vi "tsdiag_can_routine_control.vi"(6 "ATimeoutMS":i32, 8 "ARoutintID":u16, 9 "ARoutineControlType":u8, 10 "ADiagModuleIndex":i32, 11 "路径输入":path) -> (2 "返回类型":i32, 3 "路径输出":path)   [LabVIEW 2019]
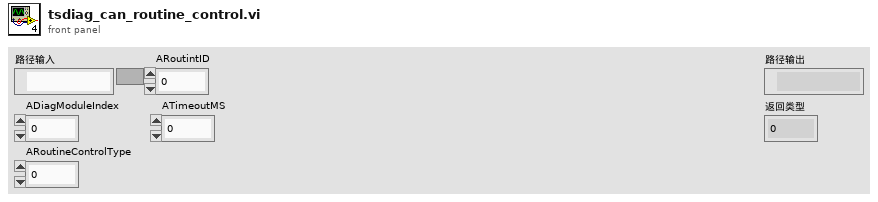
[diagram p1: front panel]
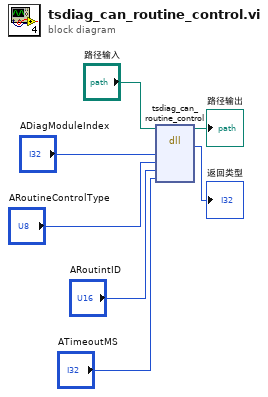
[diagram p0: block diagram]
diagram:
  n1 = dll-call lib="C:/Users/XYY/Desktop/LabView Demo/TSCAN_LB2018_V1.4_20220309/Config/TSMaster.dll" fn="tsdiag_can_routine_control"(path in="路径输入", "ADiagModuleIndex"="ADiagModuleIndex", "ARoutineControlType"="ARoutineControlType", "ARoutintID"="ARoutintID", "ATimeoutMS"="ATimeoutMS") -> (path out=→"路径输出":path, "返回类型"=→"返回类型":i32)  [unwired: 6 in, 1 out]
